vi "Update Instance VI From Target Structure.vi"(8 "tsRef":refnum<vi>, 9 "instVIref":T1, 11 "target in":refnum<class "Base Target.lvclass">) -> (3 "target out":refnum<class "Base Target.lvclass">)   [LabVIEW 2020, in "NI_TargetHelper.lvlib"]
uses:
  <vilib>/TargetSupport/NI_TargetHelper/NI_TargetHelper.lvlib
  <vilib>/TargetSupport/NI_TargetHelper/Instance VIref.ctl
  <vilib>/TargetSupport/NI_TargetHelper/Base Target/Base Target.lvclass
  704760f5-ff97-3245-97fd-fb3e0044154c.vi
  7c4268b8-172f-4f40-85f1-5527be97a933.vi
  63f2b2d2-14a6-4740-9821-b5e715b5dbbe.vi
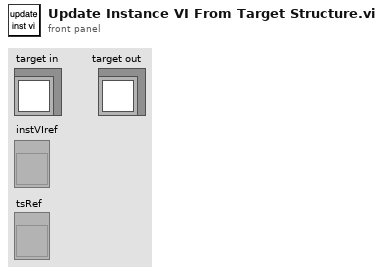
[diagram p1: front panel]
types:
  T1 = typedef "NI_TargetHelper.lvlib/Instance VIref.ctl" = refnum<vi>
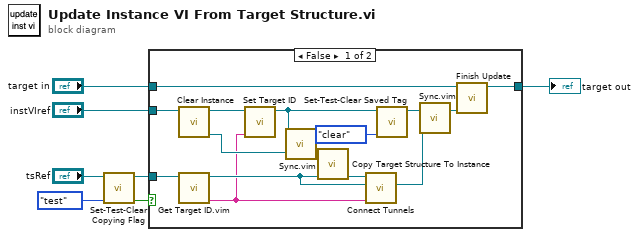
[diagram p0: block diagram]
diagram:
  n1 = call <vilib>:"Set-Test-Clear Copying Flag.vi"("op"=enum16{"test", "clear", "set"}."test", "tsRef"="tsRef") -> ("copying"=w3:bool, "tsRef out"=w4:refnum<vi>)  [unwired: 8 in]
  n2 = case shown="False" w3 {
    tunnel: "instVIref" -> [w22 _]
    tunnel: w4 -> [w18 _]
    tunnel: [w13 _] -> w2
    tunnel: "target in" -> [w8 _]
    frame False {
      n3 = call <vilib>:"Clear Instance.vi"("instVIref"=w22) -> ("diagram"=w20:refnum<vi>, "instVIref out"=w15:T1)  [unwired: 9 in]
      n4 = call "Get Target ID.vim"("ref in"=w18) -> ("target ID"=w9:string, "ref out"=w17:refnum<vi>)  [unwired: 9 in]
      n5 = call <vilib>:"Set Target ID.vi"("target ID"=w9, "instVIref"=w15) -> ("instVIref out"=w14:T1)  [unwired: 9 in]
      n6 = call "Sync.vim"("a"=w14, "b"=w20) -> ("b'"=w19:refnum<vi>)  [unwired: 24 in, 1 out]
      n7 = call <vilib>:"Copy Target Structure To Instance.vi"("tsRef"=w17, "instVI diagram"=w19) -> ("copied tsRef"=w21:refnum<vi>)  [unwired: 8 in, 1 out]
      n8 = call <vilib>:"Connect Tunnels.vi"("targetID"=w9, "orig tsRef"=w17, "inst tsRef"=w21) -> ("orig tsRef out"=w10:refnum<vi>)  [unwired: 8 in]
      n9 = call <vilib>:"Set-Test-Clear Saved Tag.vi"("op"=enum16{"test", "clear", "set"}."clear", "instVIref"=w14) -> ("instVIref out"=w12:T1)  [unwired: 8 in, 1 out]
      n10 = call "Sync.vim"("a"=w12, "b"=w10) -> ("a'"=w11:T1)  [unwired: 24 in, 1 out]
      n11 = call-dynamic "Finish Update.vi"("instVIref"=w11, "target in"=w8) -> ("target out"=w13:refnum<class "Base Target.lvclass">)  [unwired: 9 in]
    }
    frame True {
      # "this must be the target structure copied\ninto the instance VI before it has been\nremoved by scripting-- infinite recursion\nwould result if this weren't detected."
    }
  }
  "target out" <- w2
